vi "Process Live Data Q.vi"(8 "error in (no error)":errorcluster, 10 "Accel Q Elems":cluster{"output array":dbl[]}[](array[cluster]), 11 "Accelerometer in":refnum<class "Accelerometer.lvclass">) -> (0 "error out":errorcluster, 3 "Accelerometer out":refnum<class "Accelerometer.lvclass">)   [LabVIEW 2020, in "Accelerometer.lvlib" / "Accelerometer.lvclass"]
uses:
  Accelerometer.lvclass
  Accelerometer.lvclass/Accelerometer.ctl
  <vilib>/Analysis/baseanly.llb/Mean (DBL).vi
  <vilib>/Analysis/NI_AALBase.lvlib
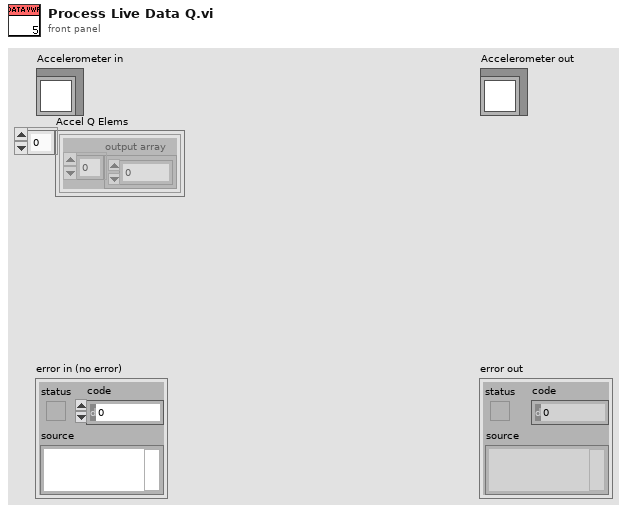
[diagram p1: front panel]
types:
  T1 = cluster{"mean":dbl, "mean":dbl, "mean":dbl, "mean":dbl}
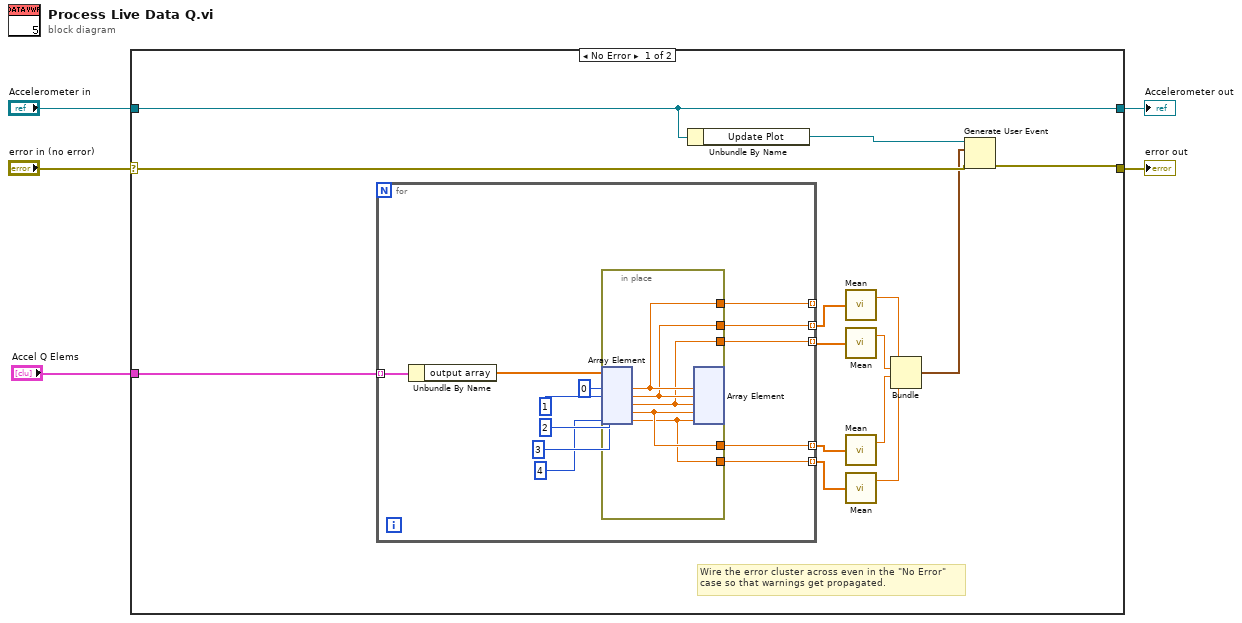
[diagram p0: block diagram]
diagram:
  n1 = case shown="No Error" "error in (no error)" {
    selector: "error in (no error)" -> [w16 w38]
    tunnel: [w15 w38] -> w4
    tunnel: [w18 w37] -> w2
    tunnel: "Accelerometer in" -> [w18 w37]
    tunnel: "Accel Q Elems" -> [w19 _]
    frame No Error {
      # "Wire the error cluster across even in the \"No Error\"\ncase so that warnings get propagated."
      n2 = for {
        tunnel: w19 -> [w26] mode=indexing
        tunnel: [w24] -> _ mode=indexing
        tunnel: [w23] -> w14 mode=indexing
        tunnel: [w22] -> w13 mode=indexing
        tunnel: [w21] -> w12 mode=indexing
        tunnel: [w20] -> w11 mode=indexing
        n3 = Unbundle By Name(w26) -> ("output array"=w25:dbl[])
        n4 = in-place {
          in-place-border: [w36] -> w24
          in-place-border: [w35] -> w23
          in-place-border: [w34] -> w22
          in-place-border: [w33] -> w21
          in-place-border: [w32] -> w20
          n5 = in-place-array #1(w25, 0, 1, 2, 3, 4) -> (w36:dbl, w35:dbl, w34:dbl, w33:dbl, w32:dbl)
          n6 = in-place-array #1(w36, w35, w34, w33, w32) -> ()  [unwired: 6 out]
        }
      }
      n7 = Unbundle By Name(w18) -> ("Update Plot"=w17:refnum<user-event>)
      n8 = call-poly <vilib>:"Mean.vi"("X"=w14) -> ("mean"=w7:dbl)  [unwired: 1 out]
      n9 = call-poly <vilib>:"Mean.vi"("X"=w13) -> ("mean"=w8:dbl)  [unwired: 1 out]
      n10 = call-poly <vilib>:"Mean.vi"("X"=w12) -> ("mean"=w10:dbl)  [unwired: 1 out]
      n11 = call-poly <vilib>:"Mean.vi"("X"=w11) -> ("mean"=w9:dbl)  [unwired: 1 out]
      n12 = Bundle("mean"=w7, "mean"=w8, "mean"=w10, "mean"=w9) -> (w6:T1)  [unwired: 1 in]
      n13 = Generate User Event(user event=w17, event data cluster=w6, error in=w16) -> (error out=w15:errorcluster)  [unwired: 1 in, 1 out]
    }
    frame Error {
    }
  }
  "error out" <- w4
  "Accelerometer out" <- w2
